vi "Tosca-Initialize Block.vi"(0 "Tosca":refnum<class "Parameters.lvclass">, 9 "block":i32, 11 "error in (no error)":errorcluster, 12 "Analysis in":T1) -> (3 "SCL":T7[](array[typedef]), 4 "Tosca out":refnum<class "Parameters.lvclass">, 10 "NumTrials":i32, 14 "Analysis out":T1, 15 "error out":errorcluster)   [LabVIEW 2020]
uses:
  Typedefs/Tosca-SCL Element.ctl
  Typedefs/Tosca-Schedule Mode.ctl
  Typedefs/Tosca-Event Type.ctl
  Typedefs/Tosca-Analysis State.ctl
  Typedefs/Tosca-Adaptation State.ctl
  Typedefs/Tosca-Adaptation Track State.ctl
  Typedefs/Tosca-Adaptation History Element.ctl
  Classes/Parameters/Histogram Data.ctl
  Classes/Parameters/Connect.ctl
  Classes/Parameters/Parameters.lvclass
  Classes/Parameters/Parameters.lvclass/Parameters.ctl
  Classes/Parameters/Read Schedule.vi
  Classes/Parameters/Read Schedule Mode.vi
  Classes/Parameters/Read Adapt.vi
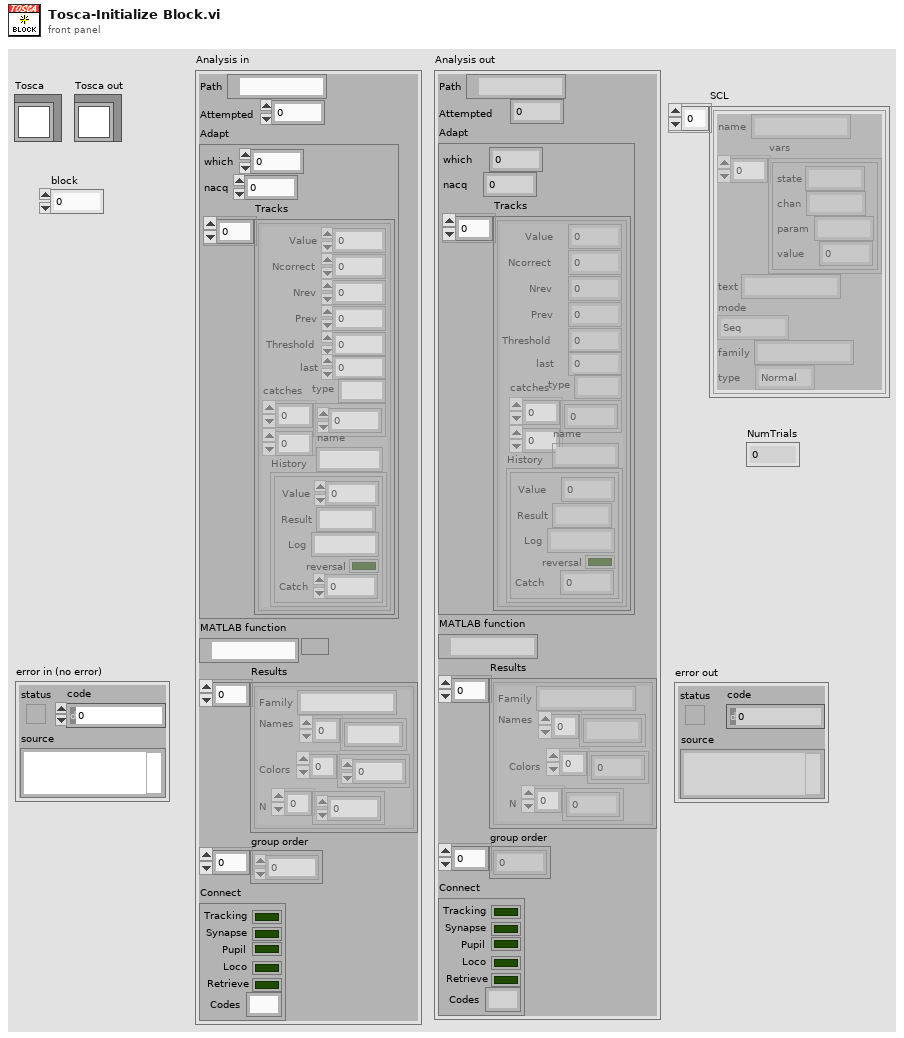
[diagram p1: front panel]
types:
  T1 = typedef "Tosca-Analysis State.ctl" = cluster{"Path":path, "Attempted":i32, "Adapt":T2, "MATLAB function":path, "Results":T5[], "group order":i32[], "Connect":T6}
  T2 = typedef "Tosca-Adaptation State.ctl" = cluster{"which":i32, "nacq":i32, "Tracks":T3[]}
  T3 = typedef "Tosca-Adaptation Track State.ctl" = cluster{"Value":dbl, "Ncorrect":i32, "Nrev":i32, "Prev":dbl, "History":T4[], "Threshold":dbl, "last":i32, "type":string, "catches":dbl[][], "name":string}
  T4 = typedef "Tosca-Adaptation History Element.ctl" = cluster{"Value":dbl, "Result":string, "Log":string, "reversal":bool, "Catch":dbl}
  T5 = typedef "Parameters.lvclass/Histogram Data.ctl" = cluster{"Family":string, "Names":string[], "Colors":u32[], "N":i32[]}
  T6 = typedef "Parameters.lvclass/Connect.ctl" = cluster{"Tracking":bool, "Synapse":bool, "Pupil":bool, "Loco":bool, "Retrieve":bool, "Codes":string}
  T7 = typedef "Tosca-SCL Element.ctl" = cluster{"name":string, "vars":cluster{"state":string, "chan":string, "param":string, "value":dbl}[], "text":string, "mode":T8, "family":string, "type":T9}
  T8 = typedef "Tosca-Schedule Mode.ctl" = enum16{"Seq", "CS+/CS-", "Adapt"}
  T9 = typedef "Tosca-Event Type.ctl" = enum16{"Normal", "CS+", "CS-"}
  T10 = typedef "Tosca-Schedule.ctl" = cluster{"Blocks":i32, "order":T11, "balance":bool, "Families":T12[], "Script":path}
  T11 = typedef "Tosca-Sequence Order.ctl" = enum16{"Sequential", "Alternate", "Randomize", "Random group", "Arbitrary"}
  T12 = typedef "Tosca-Parameter Family.ctl" = cluster{"Name":string, "Number":i32, "Vars":T13[], "Mask":bool[][], "one each":bool}
  T13 = typedef "Tosca-Parameter Table Element.ctl" = cluster{"state":string, "chan":string, "param":string, "expr":string, "dim":T14, "value":dbl[]}
  T14 = typedef "Tosca-Parameter Dimension.ctl" = enum16{"Ind", "X", "Y"}
  T15 = typedef "Tosca-Adapt.ctl" = cluster{"Switch after":i32, "Switch type":enum16{"Trials", "Reversals"}, "Tracks":T16[]}
  T16 = typedef "Tosca-Adaptive Track.ctl" = cluster{"state":string, "chan":string, "param":string, "Start":dbl, "Step":string, "Mode":enum16{"Add", "Multiply"}, "Pcatch":dbl, "Ndown":i32, "Nup":i32, "Nreverse":i32, "Min":dbl, "Max":dbl, "Catch":T17[], "do all catch":bool, "name":string, "Vars":T17[], "compute":T18, "of last":i32, "Step2":string, "after":i32}
  T17 = typedef "Tosca-Simple Variable.ctl" = cluster{"state":string, "chan":string, "param":string, "expr":string}
  T18 = typedef "Tosca-Adapt Threshold Metric.ctl" = enum16{"mean", "median"}
  T19 = cluster{"state":string, "chan":string, "param":string, "Random Element":dbl}
  T20 = cluster{"state":string, "chan":string, "param":string, "Value":dbl}
  T21 = cluster{"state":string, "chan":string, "param":string, "Value":dbl}[]
  T22 = cluster{"state":string, "chan":string, "param":string, "Numeric":dbl}
  T23 = cluster{"state":string, "chan":string, "param":string, "Numeric":dbl}[]
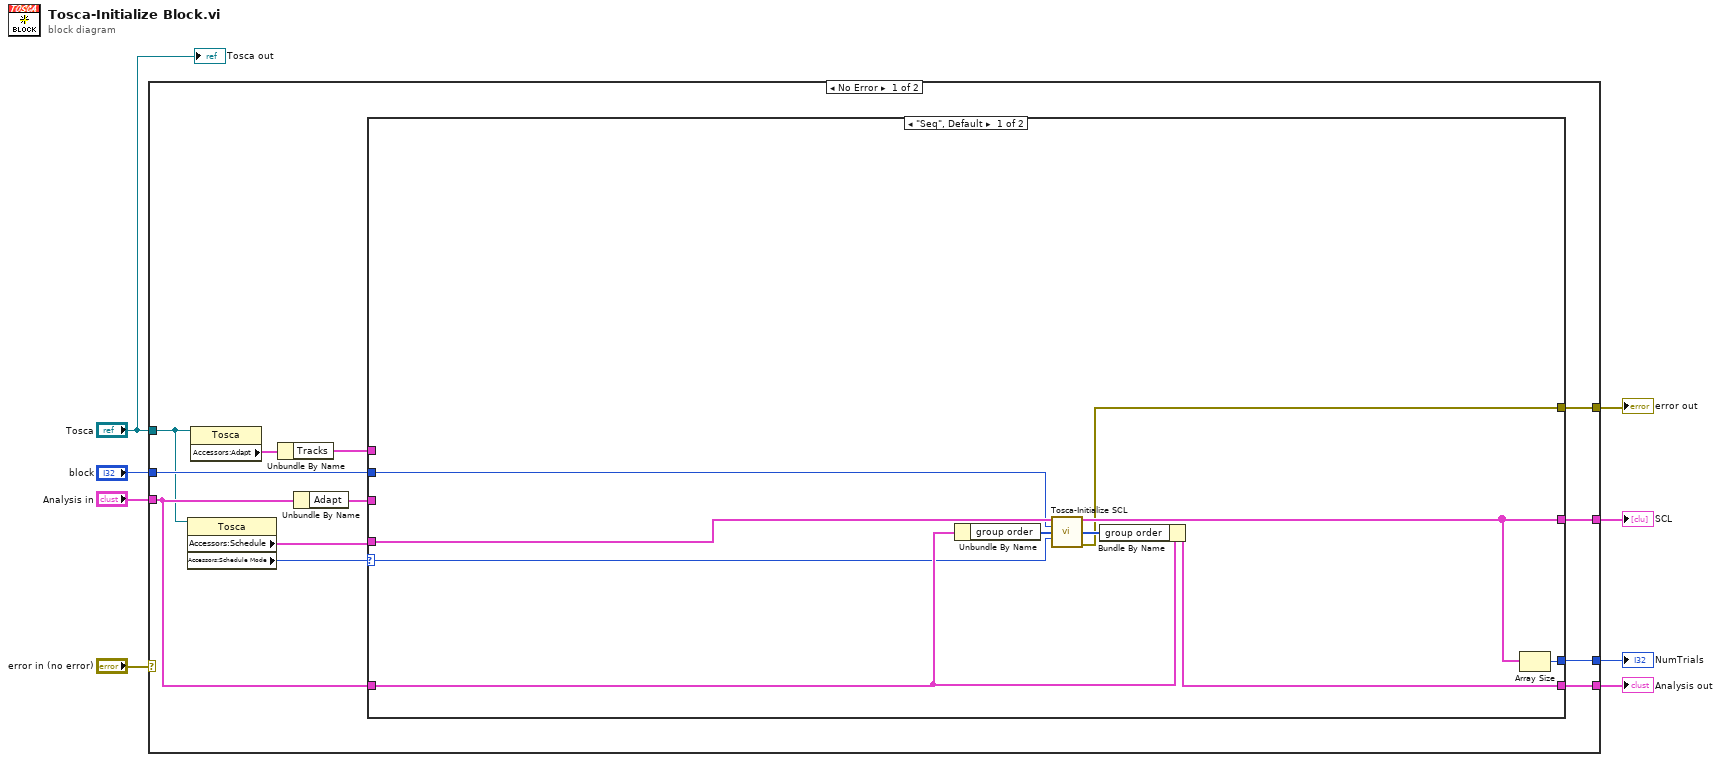
[diagram p0: block diagram]
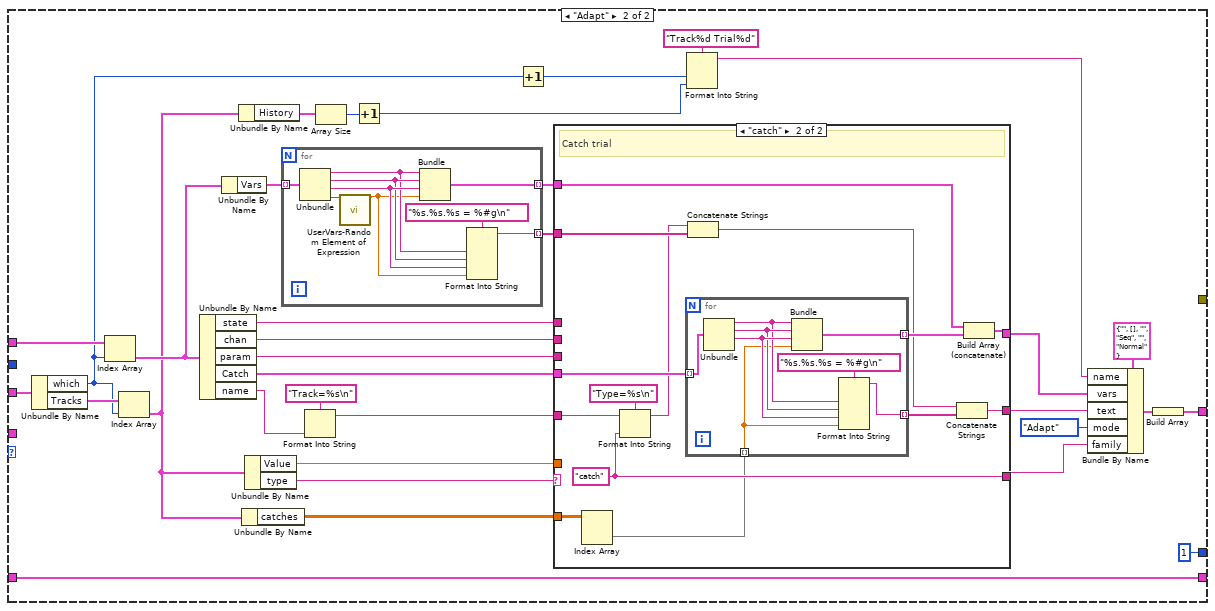
[diagram p2: hidden frame]
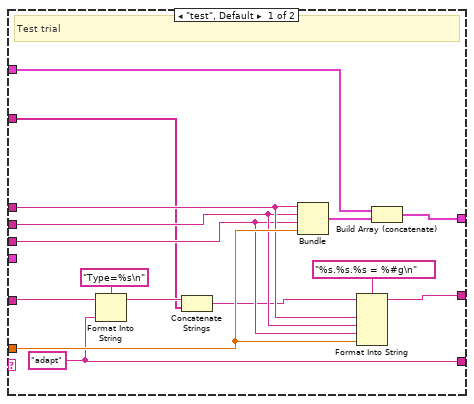
[diagram p3: hidden frame]
diagram:
  n1 = case shown="No Error" "error in (no error)" {
    selector: "error in (no error)" -> [_ w112]
    tunnel: [w20 _] -> w7
    tunnel: [w9 w112] -> w8
    tunnel: [w19 _] -> w5
    tunnel: "Analysis in" -> [w17 w111]
    tunnel: "block" -> [w18 _]
    tunnel: [w14 w111] -> w2
    tunnel: "Tosca" -> [w12 _]
    frame No Error {
      n2 = property class="Tosca"(reference=w12) -> ("Accessors:Schedule"=w11:T10, "Accessors:Schedule Mode"=w10:T8)  [unwired: 1 in, 2 out]
      n3 = property class="Tosca"(reference=w12) -> ("Accessors:Adapt"=w13:T15)  [unwired: 1 in, 2 out]
      n4 = Unbundle By Name(w13) -> ("Tracks"=w15:T16[])
      n5 = Unbundle By Name(w17) -> ("Adapt"=w16:T2)
      n6 = case shown="\"Seq\", Default" w10 {
        selector: w10 -> [w22 _]
        tunnel: w11 -> [w30 _]
        tunnel: [w28 w58] -> w20
        tunnel: [w29 1 ("NumTrials")] -> w19
        tunnel: w17 -> [w26 w31]
        tunnel: w18 -> [w25 _]
        tunnel: w16 -> [_ w48]
        tunnel: w15 -> [_ w47]
        tunnel: [w27 w31] -> w14
        tunnel: [w21 _] -> w9
        frame "Seq", Default {
          n7 = Unbundle By Name(w26) -> ("group order"=w24:i32[])
          n8 = call "Tosca-Initialize SCL.vi"("Schedule"=w30, "Block"=w25, "previous order"=w24, "Mode"=w22) -> ("SCL"=w28:T7[], "order"=w23:i32[], "error out"=w21:errorcluster)  [unwired: 9 in]
          n9 = Bundle By Name(cluster=w26, "group order"=w23) -> (w27:T1)
          n10 = Array Size(array=w28) -> (size(s)=w29:i32)
        }
        frame "Adapt" {
          n11 = Unbundle By Name(w48) -> ("which"=w36:i32, "Tracks"=w46:T3[])
          n12 = Index Array(array=w47, index=w36) -> (element=w40:T16)
          n13 = Index Array(array=w46, index=w36) -> (element=w32:T3)
          n14 = Unbundle By Name(w40) -> ("state"=w57:string, "chan"=w56:string, "param"=w55:string, "Catch"=w51:T17[], "name"=w44:string)
          n15 = Unbundle By Name(w40) -> ("Vars"=w39:T17[])
          n16 = Unbundle By Name(w32) -> ("History"=w35:T4[])
          n17 = Unbundle By Name(w32) -> ("catches"=w41:dbl[][])
          n18 = Unbundle By Name(w32) -> ("Value"=w61:dbl, "type"=w42:string)
          n19 = for {
            tunnel: w39 -> [w73] mode=indexing
            tunnel: [w71] -> w37 mode=indexing
            tunnel: [w70] -> w38 mode=indexing
            n20 = Unbundle(w73) -> ("state"=w67:string, "chan"=w68:string, "param"=w69:string, "expr"=w66:string)
            n21 = call "UserVars-Random Element of Expression.vi"("Expr"=w66) -> ("Random Element"=w65:dbl)  [unwired: 12 in, 2 out]
            n22 = Bundle("state"=w67, "chan"=w68, "param"=w69, "Random Element"=w65) -> (w70:T19)  [unwired: 1 in]
            n23 = Format Into String(format string="%s.%s.%s = %#g\n", w67, w68, w69, w65) -> (resulting string=w71:string)  [unwired: 2 in, 1 out]
          }
          n24 = Format Into String(format string="Track=%s\n", w44) -> (resulting string=w43:string)  [unwired: 2 in, 1 out]
          n25 = Array Size(array=w35) -> (size(s)=w34:i32)
          n26 = Increment(x=w34) -> (x+1=w33:i32)
          n27 = Increment(x=w36) -> (x+1=w49:i32)
          n28 = case shown="\"catch\"" w42 {
            tunnel: w61 -> [w85 _]
            tunnel: w57 -> [w83 _]
            tunnel: w56 -> [w82 _]
            tunnel: w55 -> [w81 _]
            tunnel: [w87 w93] -> w54
            tunnel: [w77 w96] -> w52
            tunnel: w51 -> [_ w102]
            tunnel: [w84 w100] -> w50
            tunnel: w43 -> [w79 w97]
            tunnel: w41 -> [_ w95]
            tunnel: w38 -> [w76 w92]
            tunnel: w37 -> [w74 w91]
            frame "test", Default {
              w77 = "adapt"
              # "Test trial"
              n29 = Format Into String(format string="Type=%s\n", initial string=w79, w77) -> (resulting string=w78:string)  [unwired: 1 in, 1 out]
              n30 = Concatenate Strings(w78, w74) -> (w75:string)
              n31 = Bundle("state"=w83, "chan"=w82, "param"=w81, "Value"=w85) -> (w88:T20)  [unwired: 1 in]
              n32 = Format Into String(format string="%s.%s.%s = %#g\n", initial string=w75, w83, w82, w81, w85) -> (resulting string=w84:string)  [unwired: 1 in, 1 out]
              n33 = Build Array (concatenate)(w76, w88) -> (w87:T21)
            }
            frame "catch" {
              w96 = "catch"
              # "Catch trial"
              n34 = Index Array(array=w95) -> (element=w94:dbl[])  [unwired: 2 in]
              n35 = Format Into String(format string="Type=%s\n", initial string=w97, w96) -> (resulting string=w90:string)  [unwired: 1 in, 1 out]
              n36 = for {
                tunnel: w102 -> [w110] mode=indexing
                tunnel: [w108] -> w101 mode=indexing
                tunnel: [w107] -> w99 mode=indexing
                tunnel: w94 -> [w103] mode=indexing
                n37 = Unbundle(w110) -> ("state"=w104:string, "chan"=w105:string, "param"=w106:string)  [unwired: 1 out]
                n38 = Bundle("state"=w104, "chan"=w105, "param"=w106, "Numeric"=w103) -> (w107:T22)  [unwired: 1 in]
                n39 = Format Into String(format string="%s.%s.%s = %#g\n", w104, w105, w106, w103) -> (resulting string=w108:string)  [unwired: 2 in, 1 out]
              }
              n40 = Concatenate Strings(w90, w91) -> (w89:string)
              n41 = Concatenate Strings(w89, w101) -> (w100:string)
              n42 = Build Array (concatenate)(w92, w99) -> (w93:T23)
            }
          }
          n43 = Format Into String(format string="Track%d Trial%d", w49, w33) -> (resulting string=w59:string)  [unwired: 2 in, 1 out]
          n44 = Bundle By Name(cluster=T7 {"name"="", "vars"=[], "text"="", "mode"=enum."Seq", "family"="", "type"=enum."Normal"} ("StimCon Element"), "name"=w59, "vars"=w54, "text"=w50, "mode"=Tosca-Schedule_Mode."Adapt", "family"=w52) -> (w62:T7)
          n45 = Build Array(w62) -> (w58:T7[])
        }
      }
    }
    frame Error {
    }
  }
  "error out" <- w8
  "SCL" <- w7
  "NumTrials" <- w5
  "Analysis out" <- w2
  "Tosca out" <- "Tosca"
